vi "DC Voltage Source (Express).vi"(9 "stop":bool, 10 "Voltage":dbl) -> (2 "error out":errorcluster)   [LabVIEW 2015]
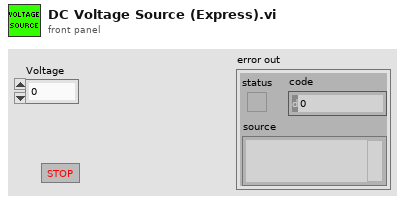
[diagram p1: front panel]
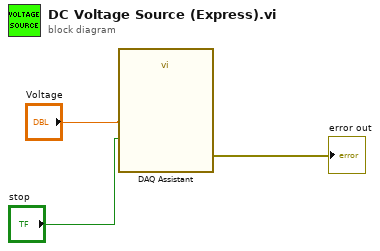
[diagram p0: block diagram]
diagram:
  n1 = call "DAQ Assistant"("data"="Voltage", "stop (T)"="stop") -> ("error out"=→"error out":errorcluster)  [unwired: 16 in, 1 out]
